vi "main_EX3.vi"   [LabVIEW 2019]
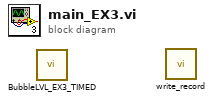
[diagram p0: block diagram]
diagram:
  n1 = call "BubbleLVL_EX3_TIMED.vi"() -> ()  [unwired: 12 in]
  n2 = call "write_record.vi"() -> ()  [unwired: 12 in]
